vi "Day 3 Puzzle 2.vi"() -> ()   [LabVIEW 2021]
uses:
  <vilib>/Utility/file.llb/Read Delimited Spreadsheet (string).vi
panel:
  out "Sum":i32
  in  "File Path":path
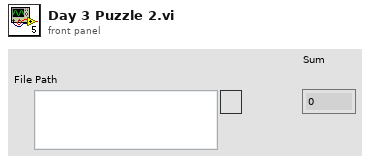
[diagram p1: front panel]
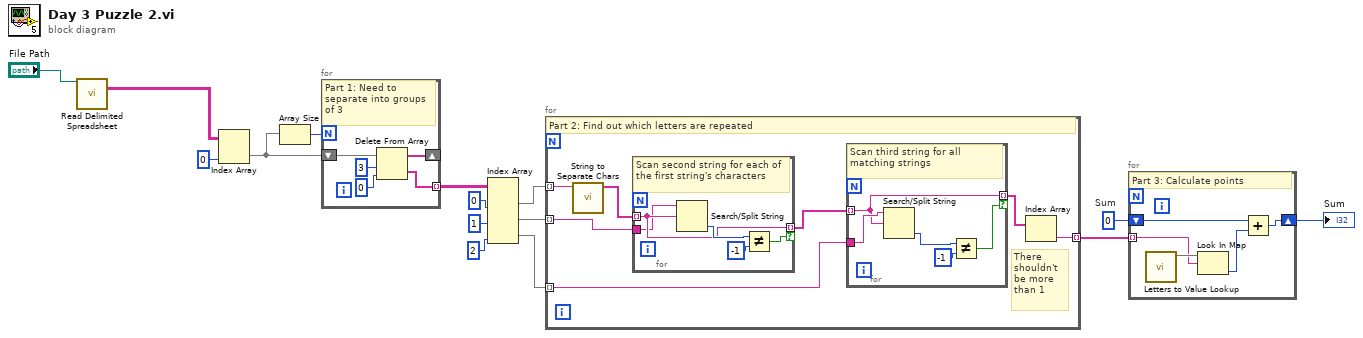
[diagram p0: block diagram]
diagram:
  w12 = 0  # Sum
  n1 = call-poly <vilib>:"Read Delimited Spreadsheet.vi"("file path (dialog if empty)"="File Path") -> ("all rows"=w1:string[][])  [unwired: 9 in, 5 out]
  n2 = Index Array(array=w1, index (col)=0 ("disabled index (col)")) -> (element=w10:string[])  [unwired: 1 in]
  n3 = Array Size(array=w10) -> (size(s)=w9:i32)
  n4 = for {
    N: w9 -> [_]
    shift-right: [w16] -> _
    shift-left: w10 -> [w20]
    tunnel: [w17] -> w8 mode=indexing
    # "Part 1: Need to separate into groups of 3"
    n5 = Delete From Array(array=w20, length=3, index=0) -> (deleted portion=w17:string[], array with subset deleted=w16:string[])
  }
  n6 = Index Array(array=w8, index (col) #1=0 ("index (row)"), index (col) #2=1 ("index (row)"), index (col) #3=2 ("index (row)")) -> (element #1=w7:string[], element #2=w6:string[], element #3=w5:string[])  [unwired: 3 in]
  n7 = for {
    tunnel: w7 -> [w27] mode=indexing
    tunnel: [w25] -> w13 mode=indexing
    tunnel: w6 -> [w24] mode=indexing
    tunnel: w5 -> [w22] mode=indexing
    # "There\nshouldn't \nbe more\nthan 1"
    # "Part 2: Find out which letters are repeated"
    n8 = call "String to Separate Chars.vi"("String"=w27) -> ("Array"=w26:string[])  [unwired: 10 in]
    n9 = for {
      tunnel: w26 -> [w29] mode=indexing
      tunnel: [w29] -> w23 mode=indexing if=w31
      tunnel: w24 -> [w28]
      # "Scan second string for each of the first string's characters"
      n10 = Search/Split String(string=w28, search string/char (-)=w29) -> (offset of match=w30:i32)  [unwired: 1 in, 2 out]
      n11 = Not Equal?(x=w30, y=-1) -> (x != y?=w31:bool)
    }
    n12 = for {
      tunnel: w23 -> [w34] mode=indexing
      tunnel: w22 -> [w35]
      tunnel: [w34] -> w21 mode=indexing if=w33
      # "Scan third string for all matching strings"
      n13 = Search/Split String(string=w35, search string/char (-)=w34) -> (offset of match=w36:i32)  [unwired: 1 in, 2 out]
      n14 = Not Equal?(x=w36, y=-1) -> (x != y?=w33:bool)
    }
    n15 = Index Array(array=w21) -> (element=w25:string)  [unwired: 1 in]
  }
  n16 = for {
    tunnel: w13 -> [w38] mode=indexing
    shift-right: [w39] -> w11
    shift-left: w12 -> [w41]
    # "Part 3: Calculate points"
    n17 = call "Letters to Value Lookup.vi"() -> ("map in"=w42:map{string, i32})  [unwired: 11 in]
    n18 = Look In Map(map=w42, key=w38) -> (value=w40:i32)  [unwired: 1 in, 1 out]
    n19 = Add(x=w41, y=w40) -> (x+y=w39:i32)
  }
  "Sum" <- w11
